vi "Get Report Settings.vi"(0 "report in":T1, 3 "error in (no error)":errorcluster) -> (6 "text color":u32(colorbox), 7 "report out":T1, 8 "text options":T2, 9 "font settings":T3, 10 "error out":errorcluster)   [LabVIEW 2020]
doc: "Retrieves information about the current font and text settings of a given report."
uses:
  <vilib>/Utility/NIReport.llb/Generate Report Object Reference.ctl
  <vilib>/Utility/NIReport.llb/NI_report.lvclass
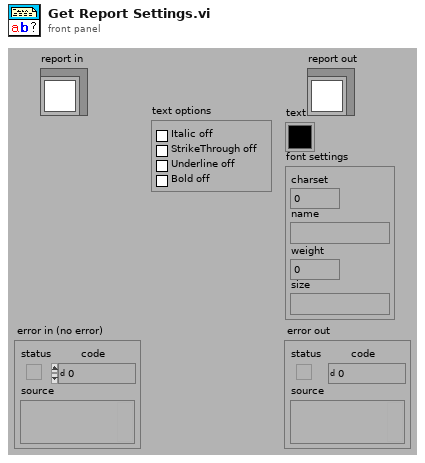
[diagram p1: front panel]
types:
  T1 = typedef "Generate Report Object Reference.ctl" = refnum<class "NI_report.lvclass">
  T2 = cluster{"Italic":bool, "StrikeThrough":bool, "Underline":bool, "Bold":bool}
  T3 = cluster{"charset":i16, "name":string, "weight":i16, "size":string}
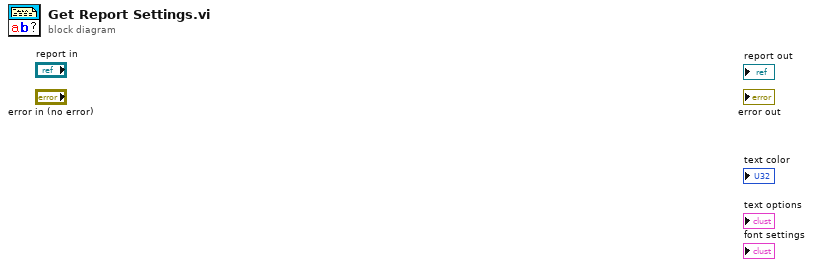
[diagram p0: block diagram]
diagram:
